vi "Listening Server Cases.vi"(7 "Listening Queue":refnum<queue>, 8 "error in (no error)":errorcluster, 9 "Data":variant, 10 "Command":string, 11 "LC Parser in":refnum<class "LC Parser.lvclass">) -> (0 "error out":errorcluster, 2 "Stop?":bool, 3 "LC Parser out":refnum<class "LC Parser.lvclass">)   [LabVIEW 2020, in "RxnRover.lvlib" / "LC Parser.lvclass"]
doc: "Case structure with messages to listen for from the control panel. If more than the basic messages need to be handled, this should be overwritten by the child class."
uses:
  LC Parser.lvclass
  LC Parser.lvclass/LC Parser.ctl
  Sub VIs/Message Queue/test Message Queue.lvlib
  Sub VIs/Message Queue/Enqueue Message (Single).vi
  Controller/Generic Plugin.lvclass
  events/Process Stopped Cluster.ctl
  RxnRover.lvlib
  C:/Users/zachc/programs/rxnrover_workspace/projects/rxnrover_exe/rxnrover/src/RxnRover/Plugin Servers/Controller/Generic Plugin.lvclass
  C:/Users/zachc/programs/rxnrover_workspace/projects/rxnrover_exe/rxnrover/src/RxnRover/Plugin Servers/LC Parser/LC Parser.lvclass
  events/New Yield Cluster.ctl
  <userlib>/RxnRover/DynamicReentrant/src/Type Defs/Message.ctl
  <userlib>/RxnRover/DynamicReentrant/Dynamic Reentrant.lvlib
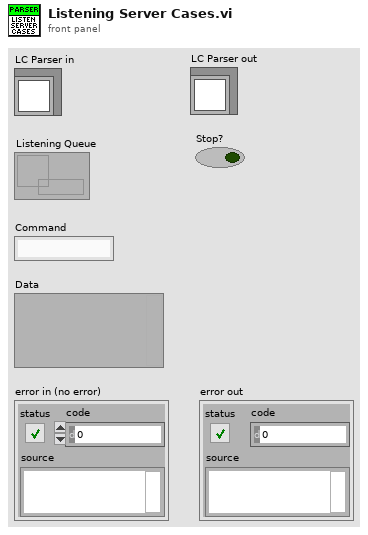
[diagram p1: front panel]
types:
  T1 = typedef "RxnRover.lvlib/New Yield Cluster.ctl" = cluster{"Name":string, "New Yield":dbl}
  T2 = typedef "RxnRover.lvlib/Process Stopped Cluster.ctl" = cluster{"Name":string, "Type":enum16{"Hardware", "Optimizer", "Analyzer"}}
  T3 = typedef "RxnRover.lvlib/LC Parser.lvclass/LC Parser State.ctl" = cluster{"Data File":path, "Last Modified":timestamp, "Peak Data":cluster{"Time Stamp":timestamp, "Peaks":string[][]}, "Yield":dbl, "New File":bool}
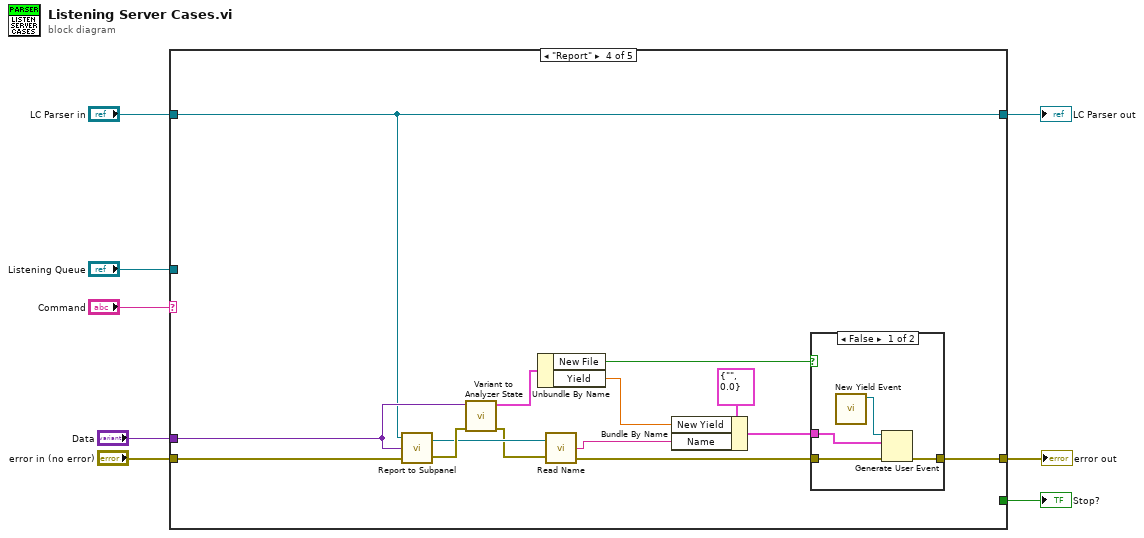
[diagram p0: block diagram]
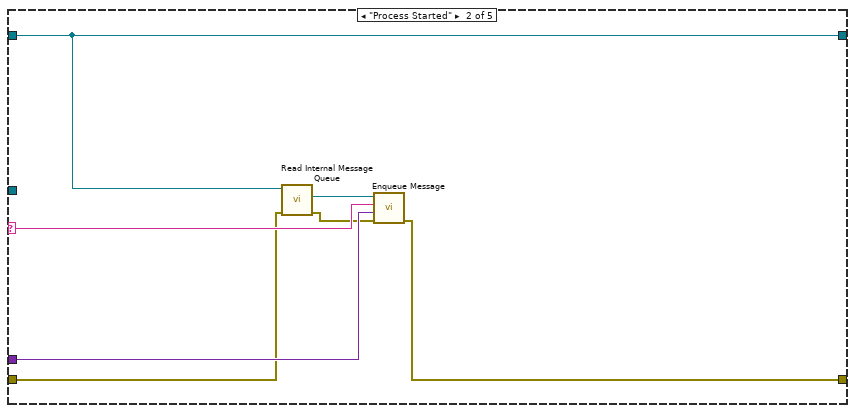
[diagram p3: hidden frame]
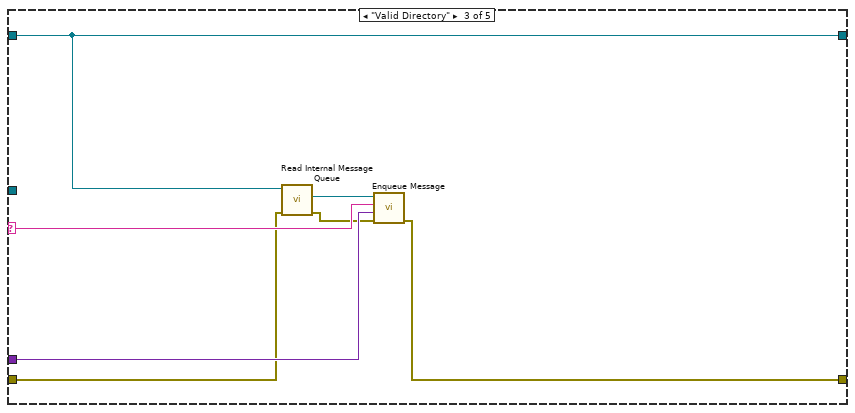
[diagram p4: hidden frame]
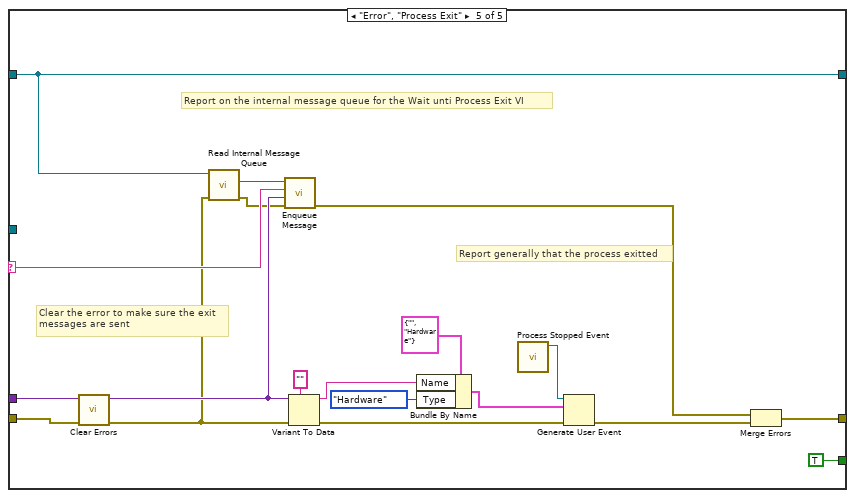
[diagram p6: hidden frame]
diagram:
  n1 = case shown="\"Report\"" "Command" {
    selector: "Command" -> [_ w17 w24 _ w52]
    tunnel: "error in (no error)" -> [w9 w11 w18 w38 w47]
    tunnel: [w9 w15 w22 w36 w50] -> w5
    tunnel: "LC Parser in" -> [w10 w13 w20 w32 w45]
    tunnel: [w10 w13 w20 w32 w45] -> w7
    tunnel: "Data" -> [_ w16 w23 w35 w51]
    tunnel: [_ _ _ _ TRUE] -> w6
    tunnel: "Listening Queue" -> [_ _ _ _ _]
    frame Default {
    }
    frame "Process Started" {
      n2 = call "Read Internal Message Queue.vi"("error in (no error)"=w11, "Generic Controller in"=w13) -> ("error out"=w12:errorcluster, "Internal Message Queue"=w14:refnum<queue>)  [unwired: 7 in, 1 out]
      n3 = call-poly "Enqueue Message.vi"("error in (no error)"=w12, "Message Data"=w16, "Message"=w17, "Message Queue"=w14) -> ("error out"=w15:errorcluster)  [unwired: 6 in, 1 out]
    }
    frame "Valid Directory" {
      n4 = call "Read Internal Message Queue.vi"("error in (no error)"=w18, "Generic Controller in"=w20) -> ("error out"=w19:errorcluster, "Internal Message Queue"=w21:refnum<queue>)  [unwired: 7 in, 1 out]
      n5 = call-poly "Enqueue Message.vi"("error in (no error)"=w19, "Message Data"=w23, "Message"=w24, "Message Queue"=w21) -> ("error out"=w22:errorcluster)  [unwired: 6 in, 1 out]
    }
    frame "Report" {
      n6 = call "Report to Subpanel.vi"("error in (no error)"=w38, "State"=w35, "controller in"=w32) -> ("error out"=w37:errorcluster, "controller out"=w31:refnum<class "LC Parser.lvclass">)
      n7 = call "Variant to Analyzer State.vi"("error in (no error)"=w37, "Message Data"=w35) -> ("error out"=w30:errorcluster, "Analyzer State"=w34:T3)  [unwired: 8 in]
      n8 = Unbundle By Name(w34) -> ("New File"=w33:bool, "Yield"=w26:dbl)
      n9 = call "Read Name.vi"("controller in"=w31, "error in (no error)"=w30) -> ("Name"=w27:string, "error out"=w29:errorcluster)  [unwired: 1 out]
      n10 = Bundle By Name(cluster=T1 {"Name"="", "New Yield"=0.0} ("Cluster"), "New Yield"=w26, "Name"=w27) -> (w25:T1)
      n11 = case shown="False" w33 {
        tunnel: w29 -> [w41 w43]
        tunnel: [w40 w43] -> w36
        tunnel: w25 -> [w39 _]
        frame False {
          n12 = call "New Yield Event.vi"() -> ("New Yield"=w42:refnum<user-event>)  [unwired: 11 in]
          n13 = Generate User Event(user event=w42, event data cluster=w39, error in=w41) -> (error out=w40:errorcluster)  [unwired: 1 in, 1 out]
        }
        frame True {
        }
      }
    }
    frame "Error", "Process Exit" {
      # "Clear the error to make sure the exit\nmessages are sent"
      # "Report generally that the process exitted"
      # "Report on the internal message queue for the Wait unti Process Exit VI"
      n14 = call <vilib>:"Clear Errors.vi"("error in (no error)"=w47) -> ("error out"=w44:errorcluster)  [unwired: 5 in, 1 out]
      n15 = call "Read Internal Message Queue.vi"("error in (no error)"=w44, "Generic Controller in"=w45) -> ("error out"=w46:errorcluster, "Internal Message Queue"=w48:refnum<queue>)  [unwired: 7 in, 1 out]
      n16 = call-poly "Enqueue Message.vi"("error in (no error)"=w46, "Message Data"=w51, "Message"=w52, "Message Queue"=w48) -> ("error out"=w49:errorcluster)  [unwired: 6 in, 1 out]
      n17 = Variant To Data(error in=w44, type="", Variant=w51) -> (data=w54:string, error out=w58:errorcluster)
      n18 = Bundle By Name(cluster=T2 {"Name"="", "Type"=enum."Hardware"} ("Process Cluster"), "Name"=w54, "Type"=enum16{"Hardware", "Optimizer"}."Hardware") -> (w55:T2)
      n19 = call "Process Stopped Event.vi"() -> ("Process Stopped"=w60:refnum<user-event>)  [unwired: 11 in]
      n20 = Generate User Event(user event=w60, event data cluster=w55, error in=w58) -> (error out=w59:errorcluster)  [unwired: 1 in, 1 out]
      n21 = Merge Errors(w49, w59) -> (w50:errorcluster)
    }
  }
  "Stop?" <- w6
  "LC Parser out" <- w7
  "error out" <- w5
